vi "Nested Actor Launcher.vi"   [LabVIEW 2020, in "Nested Actor.lvlib"]
uses:
  Nested Actor.lvlib
  Root Actor/Root Actor.lvclass
  C:/Program Files (x86)/National Instruments/LabVIEW 2020/vi.lib/ActorFramework/Actor/Actor.lvclass
  <vilib>/ActorFramework/Actor/Actor.lvclass
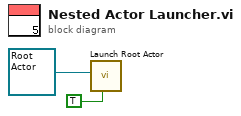
[diagram p0: block diagram]
diagram:
  n1 = call <vilib>:"Launch Root Actor.vi"("Open Actor Core front panel? (F)"=TRUE, "Actor"=refnum<class "Root Actor.lvclass"> refnum ("Nested Actor.lvlib:Root Actor.lvclass")) -> ()  [unwired: 8 in, 2 out]
